vi "Wrapper-CSM Loop.vi"   [LabVIEW 2017]
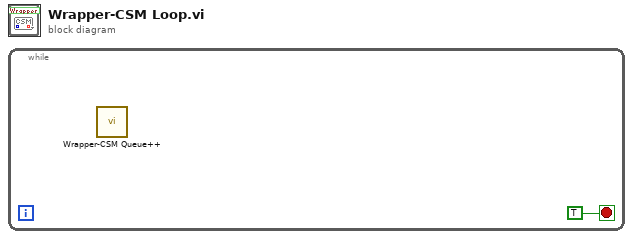
[diagram p0: block diagram]
diagram:
  n1 = while {
    stop <- TRUE stop-if-true
    n2 = call "Wrapper-CSM Queue++.vi"() -> ()  [unwired: 12 in]
  }
